vi "Handling Controller.vi"(8 "error in":errorcluster) -> ()   [LabVIEW 2015]
doc: "This VI executes continuously carrying out the current operation and responding to updates or new operations. It will often contain the timing or control code that is difficult to place directly in TeleOp. This VI generally opens all sensors and motors and isolates the rest of the robot code from knowing how the operations are carried out."
uses:
  Handling Setpoints.ctl
  Handling Operations.ctl
  Handling Published Globals.vi
  Vision/Vision Published Globals.vi
  Drive/Implementation/Drive Published Globals.vi
  Intake/Implementation/Intake Published Globals.vi
  Shooter/Implementation/Shooter Published Globals.vi
  Turret/Implementation/Turret Published Globals.vi
panel:
  in  "Distance to Motor Speed Conversions (Feet to ticks/100ms) Practice Bot":dbl[](array[numeric])=[250.0, 240.0, 210.0, 203.0, 193.0, 187.0, 190.0, 193.5, 195.0, 196.0, 197.5, 198.0, 199.0, 214.0]
  in  "Distance to Motor Speed Conversions (Feet to ticks/100ms) Comp Robot":dbl[](array[numeric])=[250.0, 240.0, 210.0, 203.0, 193.0, 187.0, 187.0, 187.0, 187.0, 187.0, 189.0, 193.0, 197.0]
  out "Current\nCmd":string="Started at  Sat 19 Mar 2016 03:48:27 PM EDT\nDefault: Reserve,  S 0.0, D 0.000000"
  # "Tip: It may be helpful to observe inputs and sensor values.\nYou may also want to display tuning or debugging controls."
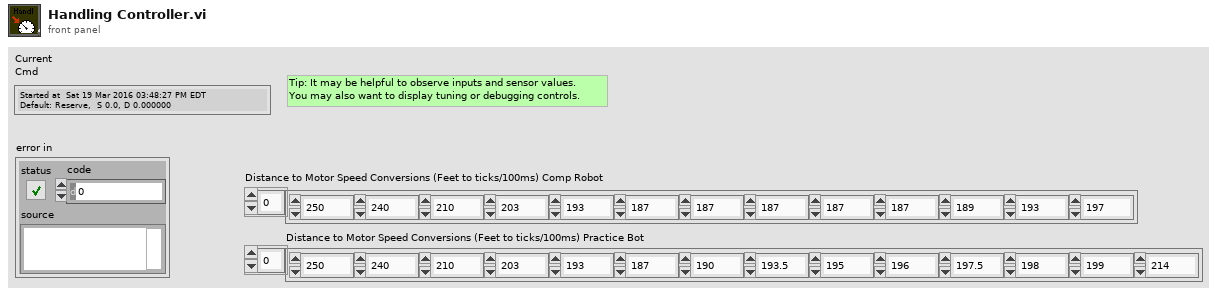
[diagram p1: front panel]
types:
  T1 = typedef "Handling Setpoints.ctl" = cluster{"Operation":T2, "Setpoint":dbl, "Duration":dbl}
  T2 = typedef "Handling Operations.ctl" = enum16{"Reserve", "Read Current", "Pickup Ball", "Fire", "Fire at Setspeed"}
  T3 = typedef "Command Status Info.ctl" = cluster{"Name":string, "Status":T4, "notifier out":T5}
  T4 = typedef "Completion Status.ctl" = enum16{"Successful", "Aborted", "Incomplete"}
  T5 = typedef "Completion Notifier.ctl" = refnum<notifier>
  T6 = cluster{"Default Command":T1, "Command Timing":cluster{"Start Time (ms)":u32, "Iterations":i32}, "Command Arguments":cluster{"Command Info":T3, "Description":string, "Default Command":T1, "notifier out":refnum<notifier>, "Subsystem Name":string}}
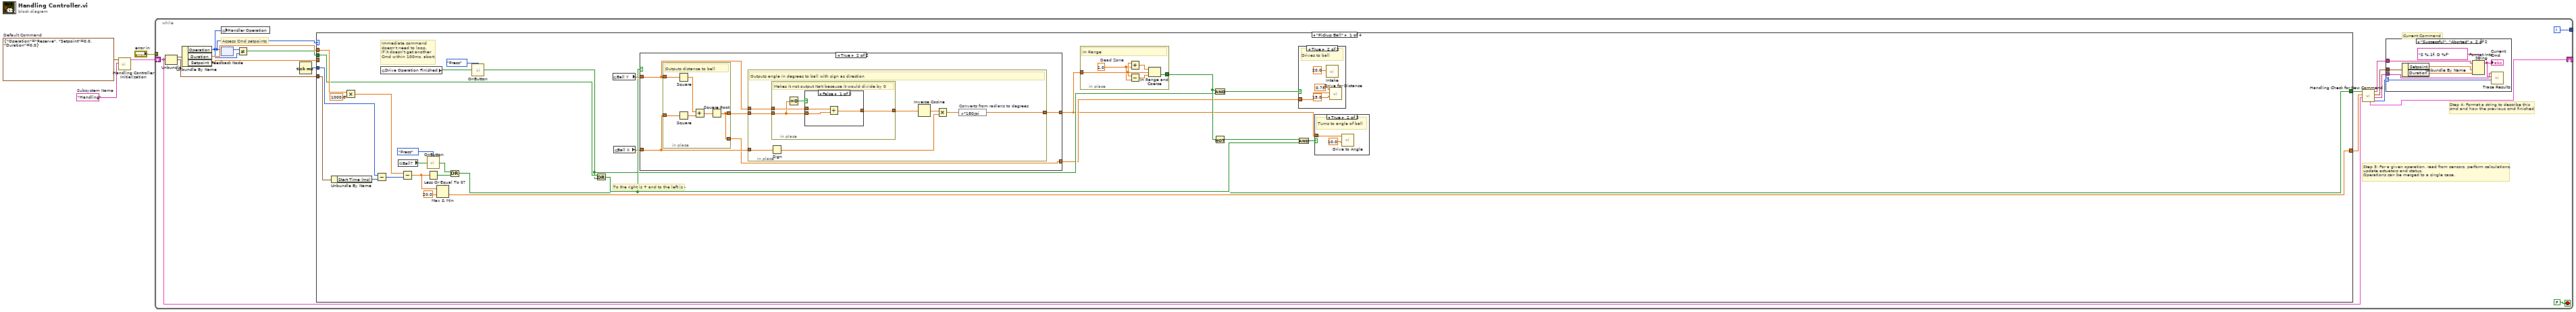
[diagram p0: block diagram]
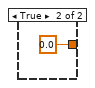
[diagram p6: hidden frame]
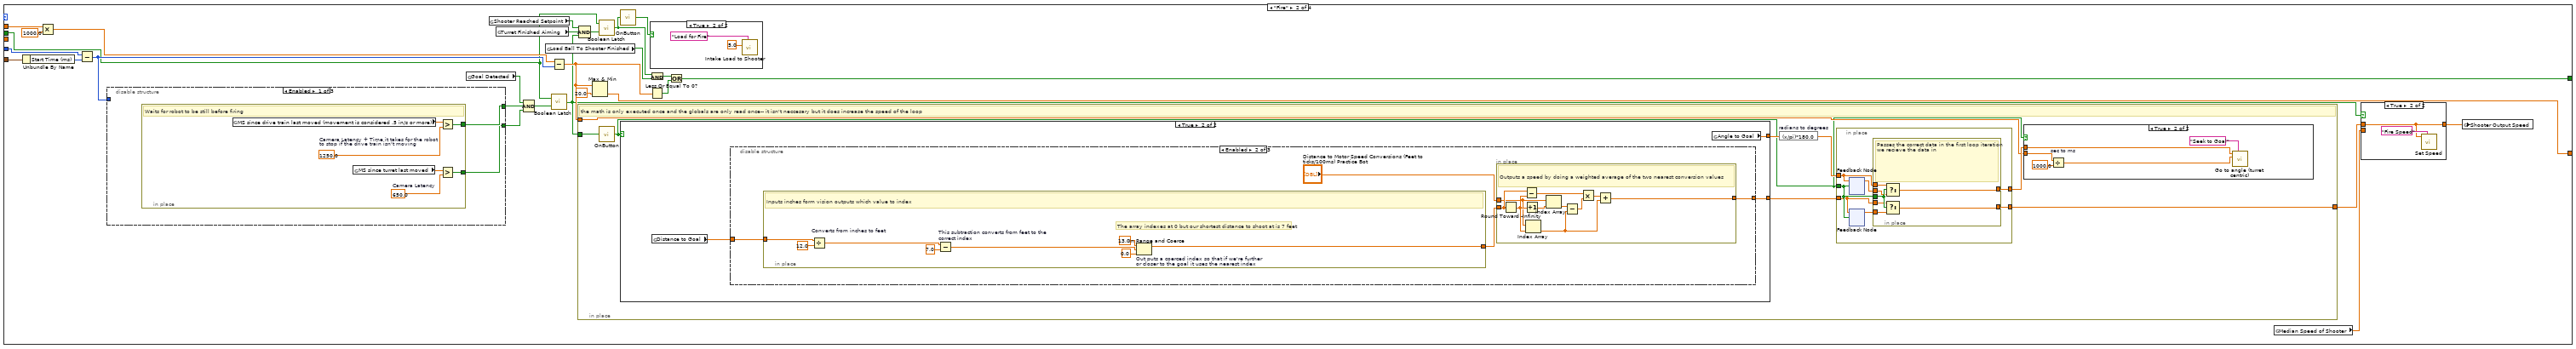
[diagram p7: hidden frame]
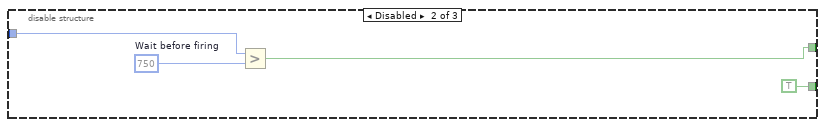
[diagram p8: hidden frame]
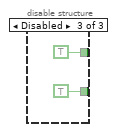
[diagram p9: hidden frame]
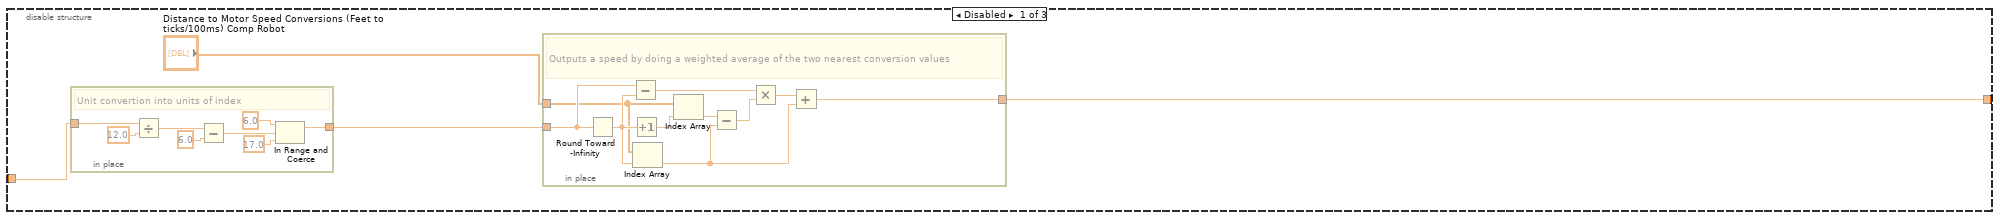
[diagram p12: hidden frame]
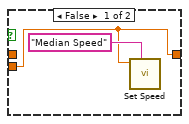
[diagram p15: hidden frame]
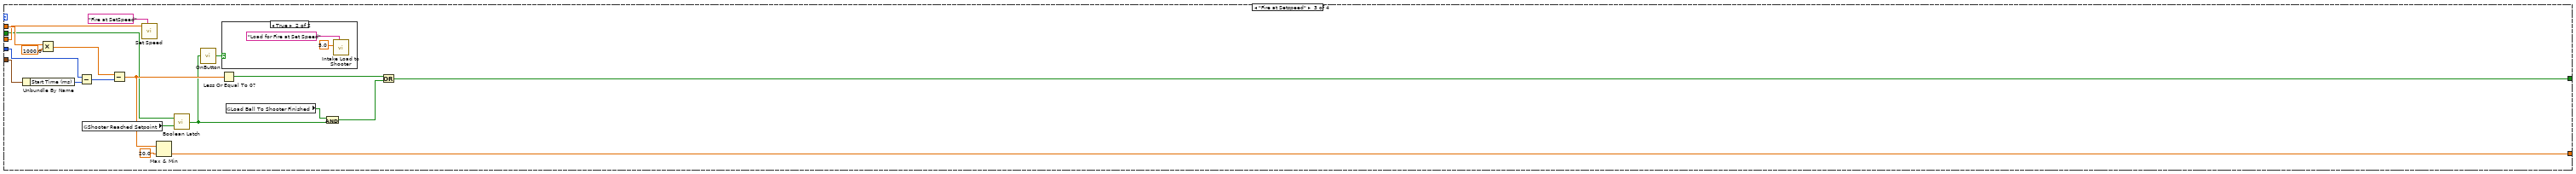
[diagram p16: hidden frame]
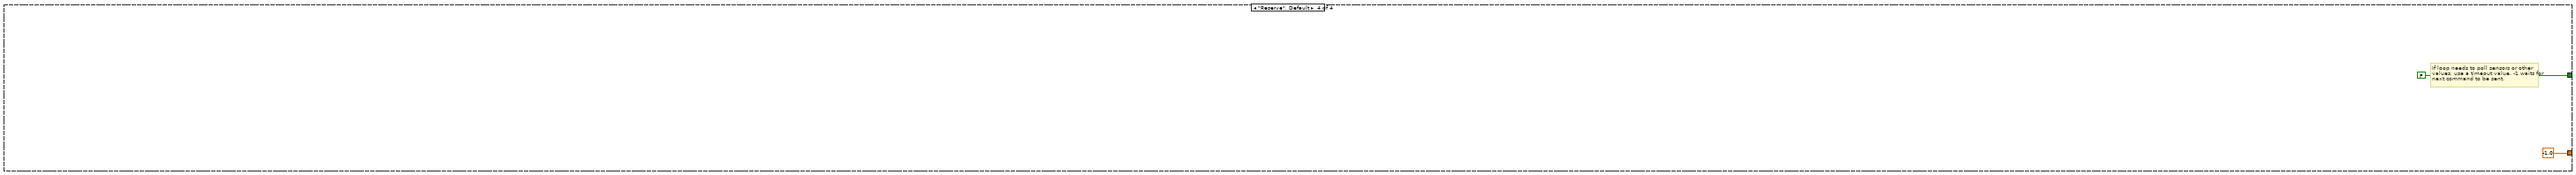
[diagram p18: hidden frame]
diagram:
  w1 = T1 {"Operation"=enum."Reserve", "Setpoint"=0.0, "Duration"=0.0}  # Default Command
  w2 = "Handling"  # Subsystem Name
  n1 = call "Handling Controller Initialization.vi"("Subsystem Name"=w2, "Default Command"=w1) -> ("Command Info"=w3:T6)  [unwired: 9 in]
  n2 = while {
    shift-right: [w14] -> _
    shift-left: w3 -> [w15]
    tunnel: [w21] -> _
    tunnel: "error in" -> [_]
    i -> [w21]
    stop <- FALSE stop-if-true
    # "Step 4: Format a string to describe this\ncmd and how the previous cmd finished"
    # "Current Command"
    # "Access Cmd setpoints"
    # "Step 3: For a given operation, read from sensors, perform calculations,\nupdate actuators and status.\nOperations can be merged to a single case."
    n3 = Unbundle(w15) -> ("Default Command"=w20:T1, "Command Timing"=w17:cluster{"Start Time (ms)":u32, "Iterations":i32})  [unwired: 1 out]
    n4 = Unbundle By Name(w20) -> ("Operation"=w5:T2, "Duration"=w19:dbl, "Setpoint"=w16:dbl)
    n5 = global write "Handling Published Globals.vi" "Handler Operation"(w5) -> ()
    n6 = feedback-in #1(w5) -> ()
    n7 = feedback #1() -> (w7:T2)  [unwired: 1 in]
    n8 = Not Equal?(x=w7, y=w5) -> (x != y?=w6:bool)
    n9 = Tick Count (ms)() -> (millisecond timer value=w18:u32)
    n10 = case shown="\"Pickup Ball\"" w5 {
      tunnel: [w50 w98 w229 -1.0] -> w12
      tunnel: [w33 w112 w223 FALSE ("ignore previous (F)")] -> w13
      tunnel: w17 -> [w54 w121 w230 _]
      tunnel: w19 -> [w52 w119 w231 _]
      tunnel: w18 -> [w53 w120 w232 _]
      tunnel: w16 -> [_ _ w227 _]
      tunnel: w6 -> [w47 w100 w221 _]
      frame "Pickup Ball" {
        # "To the right is + and to the left is -"
        # "Immediate command\ndoesn't need to loop.\nIf it doesn't get another\nCmd within 100ms, abort."
        n11 = Unbundle By Name(w54) -> ("Start Time (ms)"=w58:u32)
        n12 = Multiply(x=w52, y=1000.0) -> (x*y=w56:dbl)
        n13 = Subtract(x=w53, y=w58) -> (x-y=w55:u32)
        n14 = global read "Drive Published Globals.vi" "Drive Operation Finished"() -> (w46:bool)
        n15 = global read "Intake Published Globals.vi" "Ball?"() -> (w35:bool)
        n16 = Subtract(x=w56, y=w55) -> (x-y=w49:dbl)
        n17 = call "OnButton.vi"("Button"=w35, "Mode"=enum16{"Press", "Release", "Both"}."Press") -> ("Value"=w32:bool)
        n18 = Less Or Equal To 0?(x=w49) -> (x <= 0?=w34:bool)
        n19 = Max & Min(x=w49, y=20.0) -> (min(x,y)=w50:dbl)  [unwired: 1 out]
        n20 = Or(x=w32, y=w34) -> (x .or. y?=w33:bool)
        n21 = call "OnButton.vi"("Button"=w46, "Mode"=enum16{"Press", "Release", "Both"}."Press") -> ("Value"=w39:bool)
        n22 = Or(x=w47, y=w39) -> (x .or. y?=w42:bool)
        n23 = global read "Vision Published Globals.vi" "Ball Y"() -> (w48:dbl)
        n24 = global read "Vision Published Globals.vi" "Ball X"() -> (w44:dbl)
        n25 = case shown="True" w42 {
          tunnel: w48 -> [_ w74]
          tunnel: w44 -> [_ w72]
          tunnel: [_ w71] -> w36
          tunnel: [_ w70] -> w37
          frame False {
          }
          frame True {
            n26 = in-place {
              in-place-border: w74 -> [w77]
              in-place-border: [w75] -> w73
              in-place-border: w72 -> [w76]
              in-place-border: [w75] -> w70
              # "Outputs distance to ball"
              n27 = Square(x=w77) -> (x^2=w80:dbl)
              n28 = Square(x=w76) -> (x^2=w79:dbl)
              n29 = Add(x=w80, y=w79) -> (x+y=w78:dbl)
              n30 = Square Root ("Outputs Hypotenuse")(x=w78) -> (sqrt(x)=w75:dbl)
            }
            n31 = in-place {
              in-place-border: w74 -> [w88]
              in-place-border: w73 -> [w81]
              in-place-border: w72 -> [w86]
              in-place-border: [w82] -> w71
              # "Outputs angle in degrees to ball with sign as direction"
              n32 = Sign(1:w86) -> (0:w84:dbl)
              n33 = in-place {
                in-place-border: w88 -> [w92]
                in-place-border: [w91] -> w87
                in-place-border: w81 -> [w89]
                # "Makes it not output NaN because it would divide by 0"
                n34 = Equal To 0?(x=w89) -> (x = 0?=w90:bool)
                n35 = case shown="False" w90 {
                  tunnel: w92 -> [w95 _]
                  tunnel: w89 -> [w94 _]
                  tunnel: [w93 0.0] -> w91
                  frame False {
                    n36 = Divide(x=w95, y=w94) -> (x/y=w93:dbl)
                  }
                  frame True {
                  }
                }
              }
              n37 = Inverse Cosine(1:w87) -> (0:w85:dbl)
              n38 = Multiply(x=w85, y=w84) -> (x*y=w83:dbl)
              n39 = expression code="x*180/pi" "Converts from radians to degrees"(w83) -> (w82:dbl)
            }
          }
        }
        n40 = in-place {
          in-place-border: [w67] -> w40
          in-place-border: w36 -> [w64]
          w63 = 1.0  # Dead Zone
          # "In Range"
          n41 = Add(x=w64, y=w63) -> (x+y=w66:dbl)
          n42 = Subtract(x=w64, y=w63) -> (x-y=w65:dbl)
          n43 = In Range and Coerce(upper limit=w66, x=w64, lower limit=w65) -> (In Range?=w67:bool)  [unwired: 1 out]
        }
        n44 = And(x=w40, y=w39) -> (x .and. y?=w38:bool)
        n45 = Not(x=w40) -> (.not. x?=w41:bool)
        n46 = And(x=w41, y=w42) -> (x .and. y?=w43:bool)
        n47 = case shown="True" w38 {
          tunnel: w37 -> [_ w62]
          frame False {
          }
          frame True {
            # "Drives to ball"
            n48 = call "Intake.vi"("Duration (s)"=20.0) -> ()  [unwired: 10 in, 1 out]
            n49 = call "Drive for Distance.vi"("Duration"=15.0, "Distance (in.)"=w62, "Speed (-1 to 1)"=0.75) -> ()  [unwired: 8 in, 1 out]
          }
        }
        n50 = case shown="True" w43 {
          tunnel: w36 -> [_ w69]
          frame False {
          }
          frame True {
            # "Turns to angle of ball"
            n51 = call "Drive to Angle.vi"("Duration"=10.0, "Angle"=w69) -> ()  [unwired: 9 in, 1 out]
          }
        }
      }
      frame "Fire" {
        n52 = Unbundle By Name(w121) -> ("Start Time (ms)"=w124:u32)
        n53 = Multiply(x=w119, y=1000.0) -> (x*y=w122:dbl)
        n54 = Subtract(x=w120, y=w124) -> (x-y=w104:u32)
        n55 = disable-structure shown="Enabled" {
          disable-tunnel: [w126 w134 TRUE] -> w106
          disable-tunnel: [w125 TRUE TRUE] -> w105
          disable-tunnel: w104 -> [_ w136 _]
          frame Enabled {
            n56 = in-place {
              in-place-border: [w128] -> w126
              in-place-border: [w127] -> w125
              w129 = 650.0  # Camera Latency
              w131 = 1250.0  # Camera Latency + Time it takes for the robot to stop if the drive train isn't moving
              # "Waits for robot to be still before firing"
              n57 = global read "Drive Published Globals.vi" "MS since drive train last moved (movement is considered .5 in/s or more)"() -> (w132:dbl)
              n58 = global read "Turret Published Globals.vi" "MS since turret last moved"() -> (w130:dbl)
              n59 = Greater?(x=w132, y=w131) -> (0:w128:bool)
              n60 = Greater?(x=w130, y=w129) -> (0:w127:bool)
            }
          }
          frame Disabled {
            w135 = u32 750  # Wait before firing
            n61 = Greater?(x=w136, y=w135) -> (0:w134:bool)
          }
          frame Disabled {
          }
        }
        n62 = global read "Vision Published Globals.vi" "Goal Detected"() -> (w107:bool)
        n63 = global read "Shooter Published Globals.vi" "Shooter Reached Setpoint"() -> (w116:bool)
        n64 = global read "Turret Published Globals.vi" "Turret Finished Aiming"() -> (w114:bool)
        n65 = Compound Arithmetic op=AND(w107, w106, w105) -> (w102:bool)
        n66 = global read "Intake Published Globals.vi" "Load Ball To Shooter Finished"() -> (w111:bool)
        n67 = call "Boolean Latch.vi"("Input"=w102, "Reset"=w100) -> ("Output"=w101:bool)
        n68 = Subtract(x=w122, y=w104) -> (x-y=w117:dbl)
        n69 = in-place {
          in-place-border: w101 -> [w148]
          in-place-border: [w147] -> w109
          in-place-border: w117 -> [w145]
          # "the math is only executed once and the globals are only read once-- it isn't neccesary but it does increase the speed of the loop"
          n70 = call "OnButton.vi"("Button"=w148) -> ("Value"=w141:bool)  [unwired: 1 in]
          n71 = case shown="True" w141 {
            tunnel: [_ w163] -> w143
            tunnel: [_ w164] -> w144
            frame False {
            }
            frame True {
              n72 = global read "Vision Published Globals.vi" "Distance to Goal"() -> (w165:dbl)
              n73 = disable-structure shown="Enabled" {
                disable-tunnel: w165 -> [w168 w190 _]
                disable-tunnel: [w166 w189 _] -> w164
                frame Disabled {
                  n74 = in-place {
                    in-place-border: [w183] -> w169
                    in-place-border: w168 -> [w186]
                    # "Unit convertion into units of index"
                    n75 = Divide(x=w186, y=12.0) -> (x/y=w182:dbl)
                    n76 = Subtract(x=w182, y=6.0) -> (x-y=w180:dbl)
                    n77 = In Range and Coerce(upper limit=6.0, x=w180, lower limit=17.0) -> (coerced(x)=w183:dbl)  [unwired: 1 out]
                  }
                  n78 = in-place {
                    in-place-border: w169 -> [w178]
                    in-place-border: "Distance to Motor Speed Conversions (Feet to ticks/100ms) Comp Robot" -> [w177]
                    in-place-border: [w176] -> w166
                    # "Outputs a speed by doing a weighted average of the two nearest conversion values"
                    n79 = Round Toward -Infinity(1:w178) -> (0:w179:dbl)
                    n80 = Subtract(x=w178, y=w179) -> (x-y=w170:dbl)
                    n81 = Increment(x=w179) -> (x+1=w175:dbl)
                    n82 = Index Array(array=w177, index=w179) -> (element=w172:dbl)
                    n83 = Index Array(array=w177, index=w175) -> (element=w174:dbl)
                    n84 = Subtract(x=w174, y=w172) -> (x-y=w173:dbl)
                    n85 = Multiply(x=w170, y=w173) -> (x*y=w171:dbl)
                    n86 = Add(x=w171, y=w172) -> (x+y=w176:dbl)
                  }
                }
                frame Enabled {
                  n87 = in-place {
                    in-place-border: [w204] -> w191
                    in-place-border: w190 -> [w208]
                    # "The array indexes at 0 but our shortest distance to shoot at is 7 feet"
                    # "Inputs inches form vision outputs which value to index"
                    n88 = Divide "Converts from inches to feet"(x=w208, y=12.0) -> (x/y=w206:dbl)
                    n89 = Subtract "This subtraction converts from feet to the correct index"(x=w206, y=7.0) -> (x-y=w205:dbl)
                    n90 = In Range and Coerce "Out puts a coerced index so that if we're further or closer to the goal it uses the nearest index"(upper limit=13.0 ("lower limit"), x=w205, lower limit=0.0 ("upper limit")) -> (coerced(x)=w204:dbl)  [unwired: 1 out]
                  }
                  n91 = in-place {
                    in-place-border: w191 -> [w200]
                    in-place-border: "Distance to Motor Speed Conversions (Feet to ticks/100ms) Practice Bot" -> [w199]
                    in-place-border: [w198] -> w189
                    # "Outputs a speed by doing a weighted average of the two nearest conversion values"
                    n92 = Round Toward -Infinity(1:w200) -> (0:w201:dbl)
                    n93 = Subtract(x=w200, y=w201) -> (x-y=w192:dbl)
                    n94 = Increment(x=w201) -> (x+1=w197:dbl)
                    n95 = Index Array(array=w199, index=w201) -> (element=w194:dbl)
                    n96 = Index Array(array=w199, index=w197) -> (element=w196:dbl)
                    n97 = Subtract(x=w196, y=w194) -> (x-y=w195:dbl)
                    n98 = Multiply(x=w192, y=w195) -> (x*y=w193:dbl)
                    n99 = Add(x=w193, y=w194) -> (x+y=w198:dbl)
                  }
                }
                frame Disabled {
                }
              }
              n100 = global read "Vision Published Globals.vi" "Angle to Goal"() -> (w163:dbl)
            }
          }
          n101 = expression code="(x/pi)*180.0" "radians to degrees"(w143) -> (w142:dbl)
          n102 = in-place {
            in-place-border: w142 -> [w153]
            in-place-border: w141 -> [w155]
            in-place-border: w144 -> [w154]
            in-place-border: [w150] -> w147
            in-place-border: [w149] -> w146
            n103 = feedback #2() -> (w152:dbl)  [unwired: 1 in]
            n104 = feedback-in #2(w153, w155) -> ()
            n105 = feedback #3() -> (w151:dbl)  [unwired: 1 in]
            n106 = feedback-in #3(w154, w155) -> ()
            n107 = in-place {
              in-place-border: w155 -> [w162]
              in-place-border: w154 -> [w161]
              in-place-border: w153 -> [w160]
              in-place-border: w152 -> [w159]
              in-place-border: w151 -> [w158]
              in-place-border: [w157] -> w150
              in-place-border: [w156] -> w149
              # "Passes the correct data in the first loop iteration we recieve the data in"
              n108 = Select(t=w160, s=w162, f=w159) -> (s? t:f=w156:dbl)
              n109 = Select(t=w161, s=w162, f=w158) -> (s? t:f=w157:dbl)
            }
          }
          n110 = case shown="True" w141 {
            tunnel: w146 -> [_ w213]
            tunnel: w145 -> [_ w212]
            frame False {
            }
            frame True {
              n111 = Divide "sec to ms"(x=w212, y=1000.0 ("x")) -> (x/y=w211:dbl)
              n112 = call "Go to angle (turret centric).vi"("Description"="Seek to Goal", "Duration"=w211, "Angle (degrees)"=w213) -> ()  [unwired: 8 in, 1 out]
            }
          }
        }
        n113 = Compound Arithmetic op=AND(w116, w114, w101) -> (w99:bool)
        n114 = Max & Min(x=w117, y=20.0) -> (min(x,y)=w98:dbl)  [unwired: 1 out]
        n115 = call "Boolean Latch.vi"("Input"=w99, "Reset"=w100) -> ("Output"=w97:bool)
        n116 = call "OnButton.vi"("Button"=w97) -> ("Value"=w115:bool)  [unwired: 1 in]
        n117 = And(x=w97, y=w111) -> (x .and. y?=w110:bool)
        n118 = Less Or Equal To 0?(x=w117) -> (x <= 0?=w113:bool)
        n119 = case shown="True" w115 {
          frame False {
          }
          frame True {
            n120 = call "Intake Load to Shooter.vi"("Description"="Load for Fire", "Duration (s)"=5.0) -> ()  [unwired: 9 in, 1 out]
          }
        }
        n121 = Or(x=w110, y=w113) -> (x .or. y?=w112:bool)
        n122 = global read "Handling Published Globals.vi" "Median Speed of Shooter"() -> (w103:dbl)
        n123 = case shown="True" w101 {
          tunnel: w109 -> [_ w217]
          tunnel: [w215 w217] -> w108
          tunnel: w103 -> [w215 _]
          frame False {
            n124 = call "Set Speed.vi"("Description"="Median Speed", "Setpoint"=w215) -> ()  [unwired: 9 in, 1 out]
          }
          frame True {
            n125 = call "Set Speed.vi"("Description"="Fire Speed", "Setpoint"=w217) -> ()  [unwired: 9 in, 1 out]
          }
        }
        n126 = global write "Handling Published Globals.vi" "Shooter Output Speed"(w108) -> ()
      }
      frame "Fire at Setspeed" {
        n127 = Unbundle By Name(w230) -> ("Start Time (ms)"=w238:u32)
        n128 = Multiply(x=w231, y=1000.0) -> (x*y=w236:dbl)
        n129 = Subtract(x=w232, y=w238) -> (x-y=w233:u32)
        n130 = global read "Shooter Published Globals.vi" "Shooter Reached Setpoint"() -> (w222:bool)
        n131 = Subtract(x=w236, y=w233) -> (x-y=w234:dbl)
        n132 = call "Set Speed.vi"("Description"="Fire at SetSpeed", "Setpoint"=w227) -> ()  [unwired: 9 in, 1 out]
        n133 = Max & Min(x=w234, y=20.0) -> (min(x,y)=w229:dbl)  [unwired: 1 out]
        n134 = call "Boolean Latch.vi"("Input"=w222, "Reset"=w221) -> ("Output"=w220:bool)
        n135 = call "OnButton.vi"("Button"=w220) -> ("Value"=w225:bool)  [unwired: 1 in]
        n136 = Less Or Equal To 0?(x=w234) -> (x <= 0?=w228:bool)
        n137 = case shown="True" w225 {
          frame False {
          }
          frame True {
            n138 = call "Intake Load to Shooter.vi"("Description"="Load for Fire at Set Speed", "Duration (s)"=5.0) -> ()  [unwired: 9 in, 1 out]
          }
        }
        n139 = global read "Intake Published Globals.vi" "Load Ball To Shooter Finished"() -> (w219:bool)
        n140 = And(x=w219, y=w220) -> (x .and. y?=w224:bool)
        n141 = Or(x=w228, y=w224) -> (x .or. y?=w223:bool)
      }
      frame "Reserve", Default {
        # "If loop needs to poll sensors or other\nvalues, use a timeout value. -1 waits for\nnext command to be sent."
      }
    }
    n142 = call "Handling Check for New Command.vi"("Current Command"=w15, "Wait time (ms)"=w12, "Finished?"=w13) -> ("Completion"=w8:T4, "Subsystem Name"=w9:string, "Current Command"=w10:T1, "Initial Trace String"=w11:string, "NextCommand"=w14:T6)  [unwired: 4 in]
    n143 = case shown="\"Successful\", \"Aborted\"" w8 {
      selector: w8 -> [_ w30]
      tunnel: w11 -> [_ w26]
      tunnel: w10 -> [_ w27]
      tunnel: w9 -> [_ w23]
      frame "Incomplete", Default {
        # "Continuing current command"
      }
      frame "Successful", "Aborted" {
        # "Report and setup for next command"
        n144 = Unbundle By Name(w27) -> ("Setpoint"=w29:dbl, "Duration"=w24:dbl)
        n145 = Format Into String(format string="S %.1f, D %f", initial string=w26, w29, w24) -> (resulting string=w25:string)  [unwired: 1 in, 1 out]
        "Current\nCmd" <- w25
        n146 = call <vilib>:"Trace Results.vi"("Status of previous command"=w30, "Description"=w25, "Subsystem"=w23) -> ()  [unwired: 9 in]
      }
    }
  }
